vi "Obtain Hwnd.vi"(0 "LV DEV in":refnum<class "LV DEV.lvclass">, 11 "error in (no error)":errorcluster) -> (4 "LV DEV out":refnum<class "LV DEV.lvclass">, 15 "error out":errorcluster)   [LabVIEW 2016, in "LV DEV.lvclass"]
uses:
  LV DEV.lvclass
  D:/MDI Project/source code/Document/Child Classes/LV Doc/LV Doc.lvclass
  D:/MDI Project/source code/Document/Document.lvclass
  LV Doc.lvclass/LV Doc.ctl
  Document.lvclass/Document.ctl
  Document.lvclass
  LV Doc.lvclass
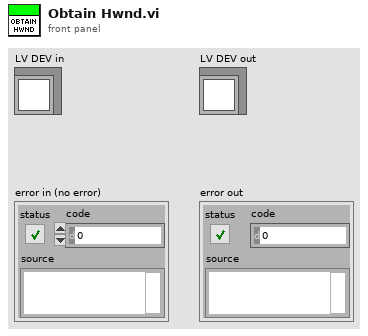
[diagram p1: front panel]
types:
  T1 = enum32{"Invalid", "Standard", "Closed", "Hidden", "Minimized", "Maximized"}
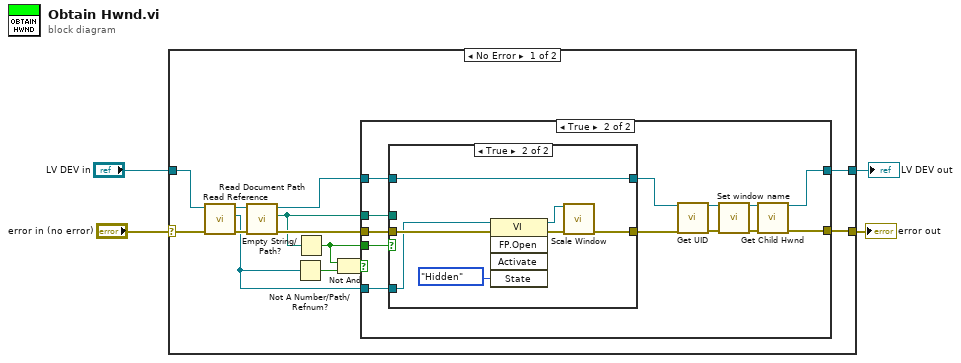
[diagram p0: block diagram]
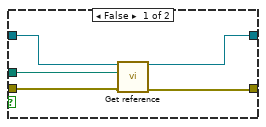
[diagram p3: hidden frame]
diagram:
  n1 = case shown="No Error" "error in (no error)" {
    selector: "error in (no error)" -> [w8 w45]
    tunnel: [w5 w45] -> w4
    tunnel: [w6 w46] -> w3
    tunnel: "LV DEV in" -> [w7 w46]
    frame No Error {
      n2 = call "Read Reference.vi"("error in (no error)"=w8, "LV Doc in"=w7) -> ("error out"=w14:errorcluster, "Reference"=w10:refnum<vi>, "LV Doc out"=w13:refnum<class "LV DEV.lvclass">)  [unwired: 7 in]
      n3 = call "Read Document Path.vi"("error in (no error)"=w14, "Document in"=w13) -> ("error out"=w16:errorcluster, "Document Path"=w15:path, "Document out"=w17:refnum<class "LV DEV.lvclass">)  [unwired: 7 in]
      n4 = Not A Number/Path/Refnum?(number/path/refnum=w10) -> (NaN/Path/Refnum?=w12:bool)
      n5 = Empty String/Path?(string/path=w15) -> (empty?=w9:bool)
      n6 = Not And(1:w12, 2:w9) -> (0:w11:bool)
      n7 = case shown="True" w11 {
        tunnel: [w18 w32] -> w6
        tunnel: [w19 w31] -> w5
        tunnel: w17 -> [w18 w21]
        tunnel: w16 -> [w19 w25]
        tunnel: w15 -> [_ w24]
        tunnel: w10 -> [_ w23]
        tunnel: w9 -> [_ w22]
        frame False {
        }
        frame True {
          n8 = case shown="True" w22 {
            tunnel: [w36 w39] -> w26
            tunnel: w25 -> [w37 w40]
            tunnel: w24 -> [w35 _]
            tunnel: w23 -> [_ w38]
            tunnel: w21 -> [w34 w44]
            tunnel: [w33 w44] -> w20
            frame False {
              n9 = call "Get reference.vi"("LV DEV.lvclass"=w34, "Vi Path"=w35, "Error in"=w37) -> ("LV DEV.lvclass"=w33:refnum<class "LV DEV.lvclass">, "Error Out"=w36:errorcluster)  [unwired: 11 in]
            }
            frame True {
              n10 = invoke class="VI" method="FP.Open"(reference=w38, error in=w40, "State"=T1."Hidden") -> (reference out=w43:refnum<vi>, error out=w42:errorcluster)  [unwired: 2 in, 3 out]
              n11 = call "Scale Window.vi"("VI in"=w43, "error in (no error)"=w42) -> ("error out"=w39:errorcluster)  [unwired: 12 in, 1 out]
            }
          }
          n12 = call "Get UID.vi"("LV Doc.lvclass"=w20, "error in (no error)"=w26) -> ("LV Doc.lvclass"=w28:refnum<class "LV DEV.lvclass">, "error out"=w29:errorcluster)  [unwired: 12 in]
          n13 = call "Set window name.vi"("LV Doc.lvclass"=w28, "error in (no error)"=w29) -> ("LV Doc.lvclass"=w27:refnum<class "LV DEV.lvclass">, "error out"=w30:errorcluster)  [unwired: 12 in]
          n14 = call "Get Child Hwnd.vi"("LV Doc.lvclass"=w27, "Error in"=w30) -> ("LV Doc.lvclass"=w32:refnum<class "LV DEV.lvclass">, "Error Out"=w31:errorcluster)  [unwired: 12 in]
        }
      }
    }
    frame Error {
    }
  }
  "error out" <- w4
  "LV DEV out" <- w3
